vi "Set startup speed.vi"(8 "error in (no error)":errorcluster, 11 "StageSPIM in":refnum<class "StageSPIM.lvclass">) -> (0 "error out":errorcluster, 3 "StageSPIM out":refnum<class "StageSPIM.lvclass">)   [LabVIEW 2012, in "StageSPIM.lvclass"]
uses:
  StageSPIM.lvclass
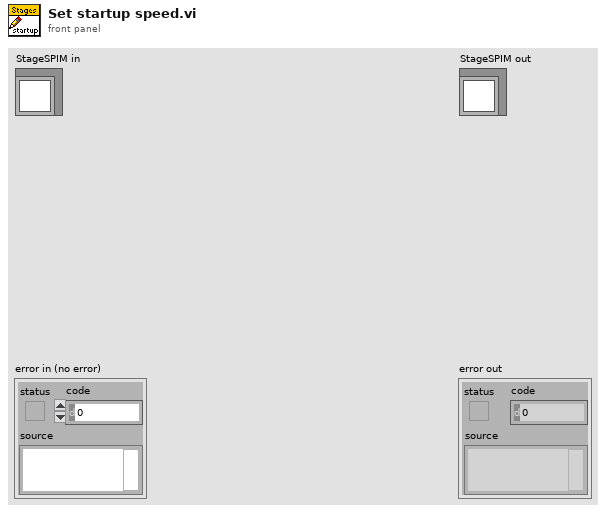
[diagram p1: front panel]
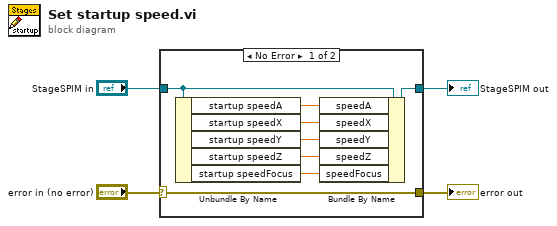
[diagram p0: block diagram]
diagram:
  n1 = case shown="No Error" "error in (no error)" {
    selector: "error in (no error)" -> [w12 w14]
    tunnel: [w12 w14] -> w3
    tunnel: [w10 w13] -> w1
    tunnel: "StageSPIM in" -> [w11 w13]
    frame No Error {
      n2 = Unbundle By Name(w11) -> ("startup speedA"=w9:dbl[unit], "startup speedX"=w8:dbl[unit], "startup speedY"=w7:dbl[unit], "startup speedZ"=w6:dbl[unit], "startup speedFocus"=w5:dbl[unit])
      n3 = Bundle By Name(cluster=w11, "speedA"=w9, "speedX"=w8, "speedY"=w7, "speedZ"=w6, "speedFocus"=w5) -> (w10:refnum<class "StageSPIM.lvclass">)
    }
    frame Error {
    }
  }
  "error out" <- w3
  "StageSPIM out" <- w1
